vi "sub_system_pause-condition.vi"(7 "cmd":enum16{"pause", "go", "read"}(ring)) -> (3 "pause":bool)   [LabVIEW 2019]
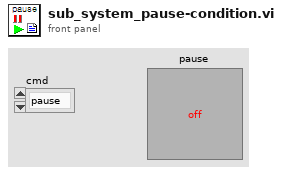
[diagram p1: front panel]
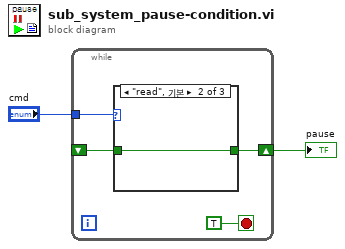
[diagram p0: block diagram]
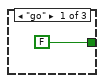
[diagram p2: hidden frame]
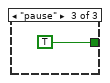
[diagram p3: hidden frame]
diagram:
  n1 = while {
    tunnel: "cmd" -> [w5]
    shift-right: [w4] -> w1
    shift-left: _ -> [w3]
    stop <- TRUE stop-if-true
    n2 = case shown="\"read\", 기본" w5 {
      tunnel: [FALSE w8 TRUE] -> w4
      tunnel: w3 -> [_ w8 _]
      frame "go" {
      }
      frame "read", Default {
      }
      frame "pause" {
      }
    }
  }
  "pause" <- w1
